vi "Dequeue Action.vi"(8 "error in (no error)":errorcluster, 11 "Queue in":refnum<queue>) -> (0 "error out":errorcluster, 1 "Data":variant, 2 "Action":T1=enum."Init", 3 "Queue out":refnum<queue>)   [LabVIEW 2019]
doc: "Dequeues the next action."
uses:
  Typedef/Scope Action.ctl
  Typedef/Message Format.ctl
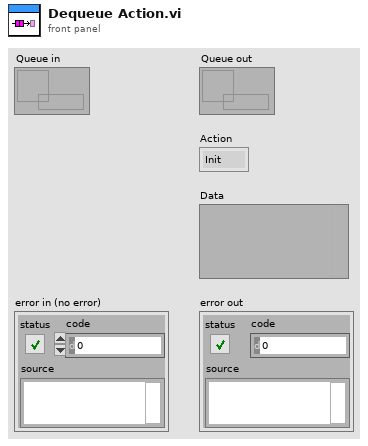
[diagram p1: front panel]
types:
  T1 = typedef "Scope Action.ctl" = enum16{"--- Driver Functions ---", "Init", "SetupV", "SetupTrigger", "SetupH", "AcquireData", "--- UI Setup ---", "Horizontal Setup", "Vertical Setup", "Trigger Setup", "--- Program Flow ---", "Error Handling", "Stop"}
  T2 = typedef "Message Format.ctl" = cluster{"Action":T1, "Data":variant}
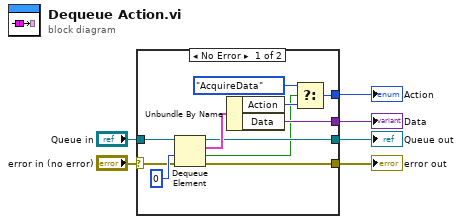
[diagram p0: block diagram]
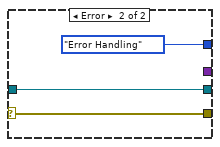
[diagram p2: hidden frame]
diagram:
  n1 = case shown="No Error" "error in (no error)" {
    selector: "error in (no error)" -> [w7 w18]
    tunnel: [w17 w18] -> w6
    tunnel: [w16 _] -> w5
    tunnel: [w13 w20] -> w4
    tunnel: "Queue in" -> [w12 w20]
    tunnel: [w10 Scope_Action."Error Handling" ("Action")] -> w2
    frame No Error {
      n2 = Dequeue Element(queue=w12, timeout in ms (-1)=0, error in (no error)=w7) -> (queue out=w13:refnum<queue>, element=w14:T2, timed out?=w9:bool, error out=w17:errorcluster)
      n3 = Unbundle By Name(w14) -> ("Action"=w15:T1, "Data"=w16:variant)
      n4 = Select(t=Scope_Action."AcquireData", s=w9, f=w15) -> (s? t:f=w10:T1)
    }
    frame Error {
    }
  }
  "error out" <- w6
  "Data" <- w5
  "Action" <- w2
  "Queue out" <- w4
